vi "Normal Inverse CDF.vi"(9 "std":dbl=1.0, 10 "mean":dbl, 11 "cdf(x)":dbl=0.5) -> (0 "error":i32, 3 "x":dbl)   [LabVIEW 2010, in "NI_Gmath.lvlib"]
doc: "Computes the continuous inverse cumulative distribution function (CDF) of the various distributions. You must manually select the polymorphic instance to use."
uses:
  NI_Gmath.lvlib
  st_error_code.ctl
panel:
  # "Normal Inverse CDF"
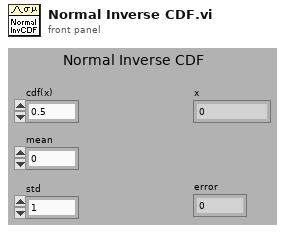
[diagram p1: front panel]
types:
  T1 = typedef "NI_Gmath.lvlib/st_error_code.ctl" = i32
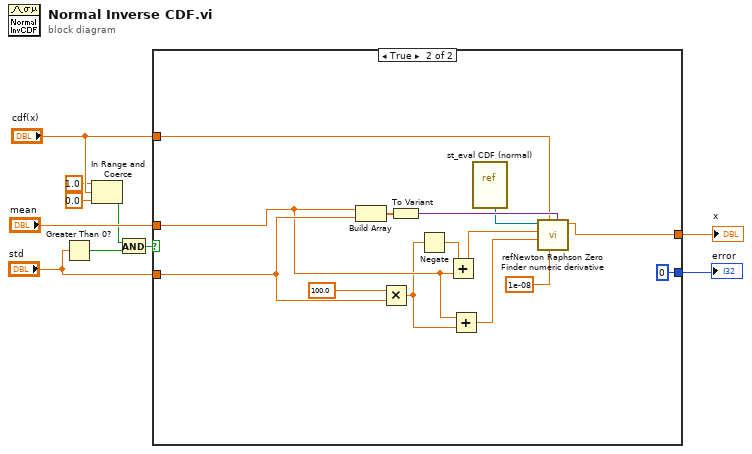
[diagram p0: block diagram]
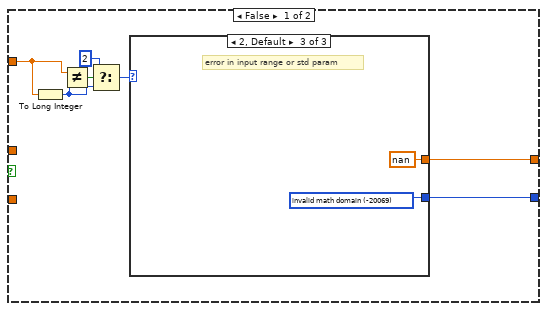
[diagram p2: hidden frame]
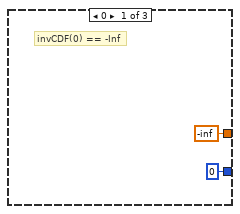
[diagram p3: hidden frame]
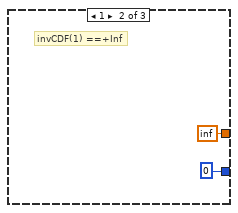
[diagram p4: hidden frame]
diagram:
  n1 = Greater Than 0?(x="std") -> (x > 0?=w2:bool)
  n2 = In Range and Coerce(upper limit=1.0, x="cdf(x)", lower limit=0.0) -> (In Range?=w3:bool)  [unwired: 1 out]
  n3 = And(x=w3, y=w2) -> (x .and. y?=w1:bool)
  n4 = case shown="True" w1 {
    tunnel: "std" -> [_ w30]
    tunnel: [w16 0 ("invalid math domain")] -> w9
    tunnel: [w17 w34] -> w8
    tunnel: "cdf(x)" -> [w14 w32]
    tunnel: "mean" -> [_ w26]
    frame False {
      n5 = To Long Integer(number=w14) -> (32bit integer=w13:i32)
      n6 = Not Equal?(x=w14, y=w13) -> (x != y?=w15:bool)
      n7 = Select(t=2, s=w15, f=w13) -> (s? t:f=w12:i32)
      n8 = case shown="2, Default" w12 {
        tunnel: [-inf inf nan] -> w17
        tunnel: [0 ("invalid math domain") 0 ("invalid math domain") w22] -> w16
        frame 0 {
          # "invCDF(0) == -Inf"
        }
        frame 1 {
          # "invCDF(1) ==+Inf"
        }
        frame 2, Default {
          w22 = T1 -20069 items=["invalid math domain"=-20069, "Fourier interpolation size m >= n"=-20070, "empty array"=-20003] ("stat interp error code")
          # "error in input range or std param"
        }
      }
    }
    frame True {
      n9 = Build Array(w26, w30) -> (w36:dbl[])
      n10 = Multiply(x=100.0, y=w30) -> (x*y=w25:dbl)
      n11 = To Variant(anything=w36) -> (Variant=w35:variant)
      n12 = Negate(x=w25) -> (-x=w28:dbl)
      n13 = Add(x=w28, y=w26) -> (x+y=w27:dbl)
      n14 = Add(x=w26, y=w25) -> (x+y=w24:dbl)
      n15 = vi-ref "st_eval CDF (normal).vi"() -> ("vi reference"=w33:refnum<vi>)
      n16 = call "refNewton Raphson Zero Finder numeric derivative.vi"("function parameters"=w35, "accuracy"=1e-08, "level"=w32, "end"=w24, "start"=w27, "function refnum"=w33) -> ("zero"=w34:dbl)  [unwired: 2 in, 3 out]
    }
  }
  "x" <- w8
  "error" <- w9
